vi "merge one reactor.vi"(7 "merge_preexisting":bool, 8 "error in (no error)":errorcluster, 9 "current_starttime":i32, 10 "simulation_starttime":i32, 11 "working_dir":string) -> (0 "error out":errorcluster)   [LabVIEW 2019, in "libFileFunctions.lvlib"]
doc: "void merge_one_reactor(const char* working_dir, int simulation_starttime, int current_starttime, bool merge_preexisting);"
uses:
  libFileFunctions.lvlib
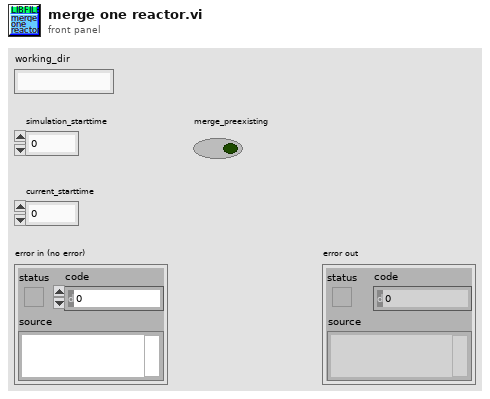
[diagram p1: front panel]
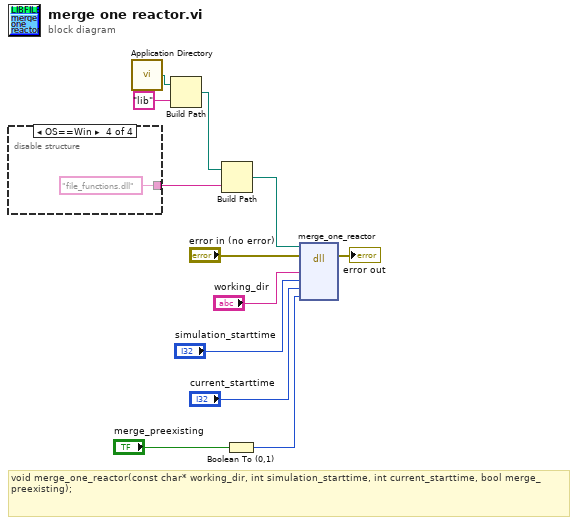
[diagram p0: block diagram]
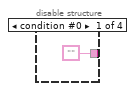
[diagram p2: hidden frame]
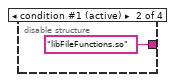
[diagram p3: hidden frame]
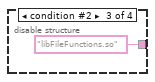
[diagram p4: hidden frame]
diagram:
  # "void merge_one_reactor(const char* working_dir, int simulation_starttime, int current_starttime, bool merge_preexisting);"
  n1 = disable-structure shown="OS==Win" {
    disable-tunnel: ["" "libFileFunctions.so" ("name or relative path") "libFileFunctions.so" ("name or relative path") "file_functions.dll" ("name or relative path")] -> w2
    frame condition #0 {
    }
    frame condition #1 (active) {
    }
    frame condition #2 {
    }
    frame condition #3 {
    }
  }
  n2 = call <vilib>:"Application Directory.vi"() -> ("Application Directory"=w5:path)
  n3 = Build Path(base path=w5, name or relative path="lib") -> (appended path=w3:path)
  n4 = Build Path(base path=w3, name or relative path=w2) -> (appended path=w1:path)
  n5 = Boolean To (0,1)(Boolean="merge_preexisting") -> (0, 1=w8:i16)
  n6 = dll-call lib="home/paul/Schreibtisch/Biogas_plant_setup/LabView/lib/libFileFunctions/libFileFunctions.*" fn="merge_one_reactor"(path in=w1, error in="error in (no error)", "working_dir"="working_dir", "simulation_starttime"="simulation_starttime", "current_starttime"="current_starttime", "merge_preexisting"=w8) -> (error out=→"error out":errorcluster)  [unwired: 6 in, 1 out]
